vi "Bundle Script_Properties Remove.vi"(8 "error in":errorcluster, 9 "Remove Indices":i32[](array[numeric]), 10 "Property Array":T2(array[cluster]), 11 "Affected Items":T1) -> (0 "error out":errorcluster, 2 "Objects":refnum<vi>[](array[refnum]))   [LabVIEW 2023]
doc: "Take Tag array OR index array and remove items."
uses:
  top/BundleMagic.ctl
panel:
  # "OR"
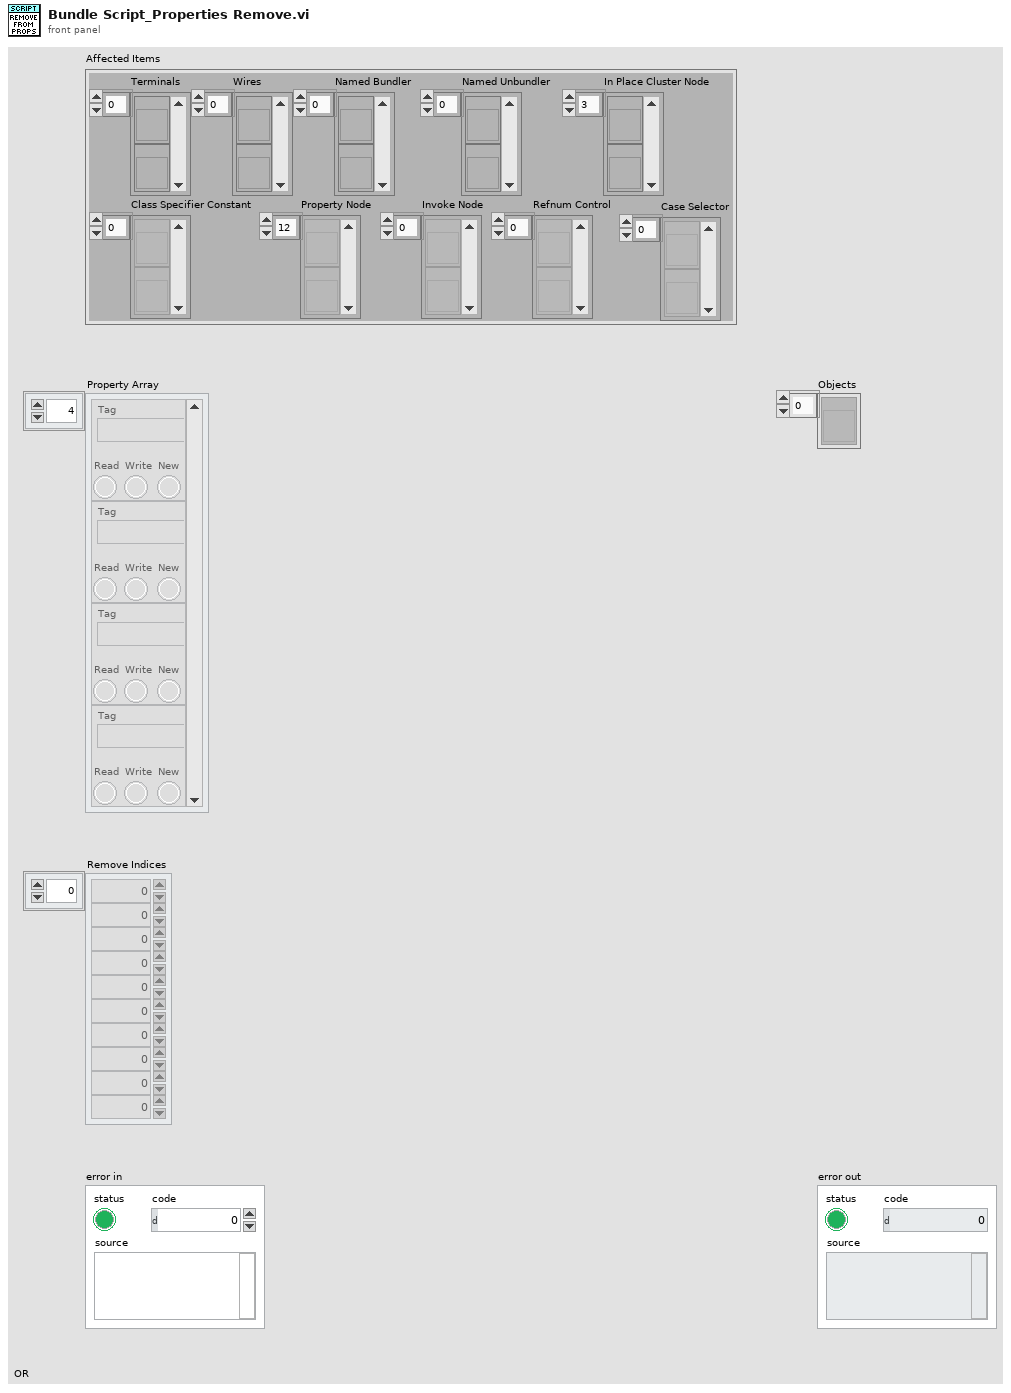
[diagram p1: front panel]
types:
  T1 = typedef "BundleMagic.ctl" = cluster{"Terminals":refnum<vi>[], "Wires":refnum<vi>[], "Named Bundler":refnum<vi>[], "Named Unbundler":refnum<vi>[], "In Place Cluster Node":refnum<vi>[], "Class Specifier Constant":refnum<vi>[], "Property Node":refnum<vi>[], "Invoke Node":refnum<vi>[], "Refnum Control":refnum<vi>[], "Case Selector":refnum<vi>[]}
  T2 = cluster{"Tag":string, "Read":bool, "Write":bool, "New":bool}[]
  T3 = cluster{"Index":u16, "Property Type":enum16{"Unknown", "Base", "Scripting", "Private", "Deprecated", "None", "Divider"}, "ID String":string, "Dotted ID String":string, "Class":string, "Parent":string, "Display name full":string, "Display name short":string, "Parents Array":string[], "Indent":u16}
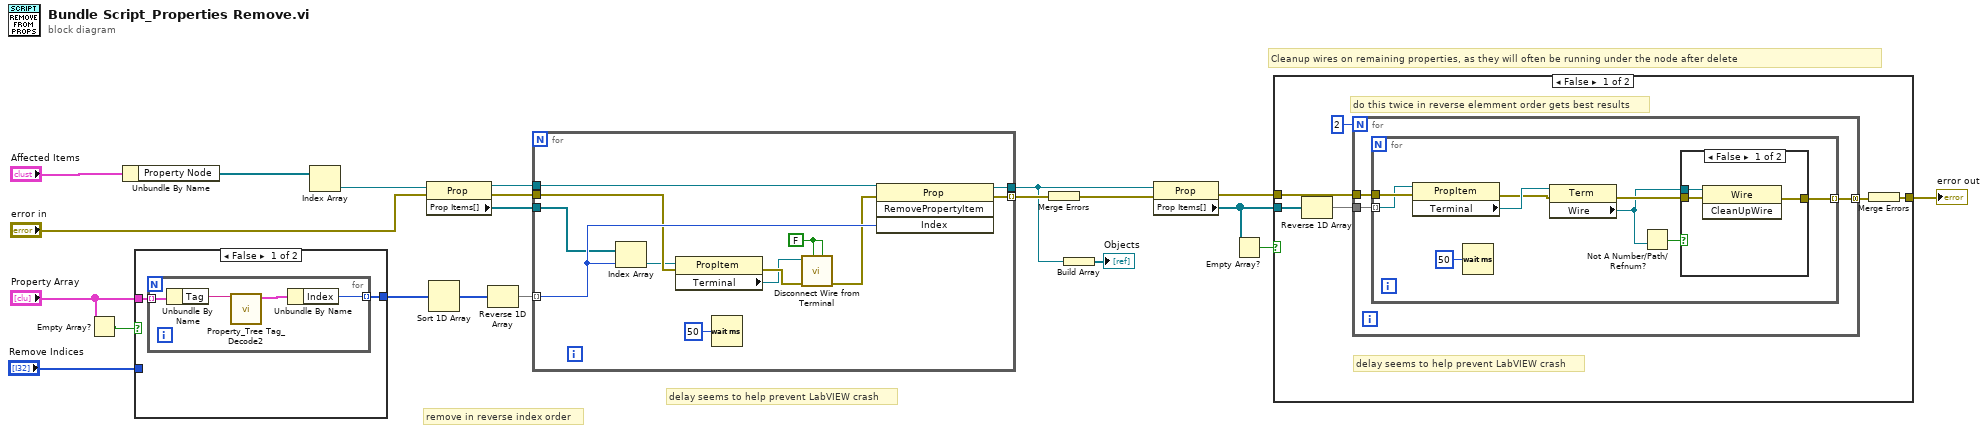
[diagram p0: block diagram]
diagram:
  # "delay seems to help prevent LabVIEW crash"
  # "Cleanup wires on remaining properties, as they will often be running under the node after delete"
  # "remove in reverse index order"
  n1 = Empty Array?(array="Property Array") -> (empty?=w2:bool)
  n2 = Unbundle By Name("Affected Items") -> ("Property Node"=w19:refnum<vi>[])
  n3 = case shown="False" w2 {
    tunnel: "Property Array" -> [w23 _]
    tunnel: [w22 w28] -> w11
    tunnel: "Remove Indices" -> [_ w28]
    frame False {
      n4 = for {
        tunnel: w23 -> [w27] mode=indexing
        tunnel: [w25] -> w22 mode=indexing
        n5 = Unbundle By Name(w27) -> ("Tag"=w24:string)
        n6 = call "Property_Tree Tag_Decode2.vi"("Tag In"=w24) -> ("TagData"=w26:T3)  [unwired: 10 in]
        n7 = Unbundle By Name(w26) -> ("Index"=w25:u16)
      }
    }
    frame True {
    }
  }
  n8 = Index Array(array=w19) -> (element=w7:refnum<vi>)  [unwired: 1 in]
  n9 = property class="Prop"(reference=w7, error in="error in") -> (reference out=w14:refnum<vi>, error out=w13:errorcluster, "Prop Items[]"=w12:refnum<vi>[])
  n10 = Sort 1D Array(array=w11) -> (sorted array=w16:i32[])
  n11 = Reverse 1D Array(array=w16) -> (reversed array=w15:i32[])
  n12 = for {
    tunnel: w15 -> [w40] mode=indexing
    tunnel: w14 -> [w39]
    tunnel: w13 -> [w38]
    tunnel: w12 -> [w37]
    tunnel: [w36] -> w18 mode=indexing
    tunnel: [w35] -> w10
    w34 = FALSE ("Clean Up wire")
    n13 = Index Array(array=w37, index=w40) -> (element=w31:refnum<vi>)
    n14 = property class="PropItem"(reference=w31, error in=w38) -> (error out=w33:errorcluster, "Terminal"=w30:refnum<vi>)  [unwired: 1 out]
    n15 = Wait (ms)(milliseconds to wait=u32 50) -> ()  [unwired: 1 out]
    n16 = call "Disconnect Wire from Terminal.vi"("Remove Loose Ends"=w34, "Clean Up wire"=w34, "error in"=w33, "Terminal in"=w30) -> ("error out"=w32:errorcluster)  [unwired: 3 in, 4 out]
    n17 = invoke class="Prop" method="RemovePropertyItem"(reference=w39, error in=w32, "Index"=w40) -> (reference out=w35:refnum<vi>, error out=w36:errorcluster)  [unwired: 1 in, 2 out]
  }
  n18 = Merge Errors(w18) -> (w9:errorcluster)
  n19 = Build Array(w10) -> (→"Objects":refnum<vi>[])
  n20 = property class="Prop"(reference=w10, error in=w9) -> (error out=w8:errorcluster, "Prop Items[]"=w5:refnum<vi>[])  [unwired: 1 out]
  n21 = Empty Array?(array=w5) -> (empty?=w4:bool)
  n22 = case shown="False" w4 {
    tunnel: w5 -> [w46 _]
    tunnel: w8 -> [w45 w63]
    tunnel: [w43 w63] -> w6
    frame False {
      # "do this twice in reverse elemment order gets best results"
      # "delay seems to help prevent LabVIEW crash"
      n23 = Reverse 1D Array(array=w46) -> (reversed array=w42:refnum<vi>[])
      n24 = for {
        N: 2 -> [_]
        tunnel: w45 -> [w49]
        tunnel: [w48] -> w44 mode=concatenating
        tunnel: w42 -> [w47]
        n25 = for {
          tunnel: w47 -> [w57] mode=indexing
          tunnel: w49 -> [w58]
          tunnel: [w53] -> w48 mode=indexing
          n26 = property class="PropItem"(reference=w57, error in=w58) -> (error out=w55:errorcluster, "Terminal"=w56:refnum<vi>)  [unwired: 1 out]
          n27 = Wait (ms)(milliseconds to wait=u32 50) -> ()  [unwired: 1 out]
          n28 = property class="Term"(reference=w56, error in=w55) -> (error out=w54:errorcluster, "Wire"=w52:refnum<vi>)  [unwired: 1 out]
          n29 = Not A Number/Path/Refnum?(number/path/refnum=w52) -> (NaN/Path/Refnum?=w51:bool)
          n30 = case shown="False" w51 {
            tunnel: w52 -> [w61 _]
            tunnel: w54 -> [w60 w62]
            tunnel: [w59 w62] -> w53
            frame False {
              n31 = invoke class="Wire" method="CleanUpWire"(reference=w61, error in=w60) -> (error out=w59:errorcluster)  [unwired: 1 in, 2 out]
            }
            frame True {
            }
          }
        }
      }
      n32 = Merge Errors(w44) -> (w43:errorcluster)
    }
    frame True {
    }
  }
  "error out" <- w6
